vi "DSF.Engine.Interface.Builder.Read.Response.vi"(8 "error in (no error)":errorcluster, 9 "timeout in ms (0)":i32 format="%d ms", 11 "Builder Interface in":refnum<class "DSF.Engine.Interface.Builder.lvclass">) -> (0 "error out":errorcluster, 1 "empty?":bool, 2 "response":T1, 3 "Builder Interface out":refnum<class "DSF.Engine.Interface.Builder.lvclass">, 4 "# elements":u32)   [LabVIEW 2017, in "DSF.Engine.lvlib" / "DSF.Engine.Interface.Builder.lvclass"]
uses:
  DSF.Engine.Interface.Builder.lvclass
  C:/github/data-sharing-framework/dsf core/Source/Engine/Classes/Interface/DSF.Engine.Interface.lvclass
  DSF.Engine.Interface.Builder.Response Data.ctl
  DSF.Engine.Interface.Builder.Response.ctl
  DSF.Engine.Interface.lvclass/DSF.Engine.Interface.ctl
  Debug/DSF.Engine.Debug Flags.FIFO.lvclass/DSF.Engine.Debug Flags.FIFO.ctl
  Debug/DSF.Engine.Debug Flags.FIFO.Get Infinite Timeouts.vi
  Debug/DSF.Engine.Debug Flags.FIFO.lvclass
  DSF.Engine.Interface.lvclass
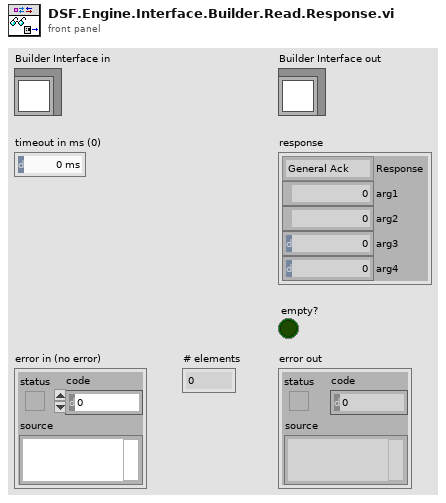
[diagram p1: front panel]
types:
  T1 = typedef "DSF.Engine.lvlib/DSF.Engine.Interface.Builder.lvclass/DSF.Engine.Interface.Builder.Response Data.ctl" = cluster{"Response":T2, "arg1":i32, "arg2":i32, "arg3":i32, "arg4":i32}
  T2 = typedef "DSF.Engine.lvlib/DSF.Engine.Interface.Builder.lvclass/DSF.Engine.Interface.Builder.Response.ctl" = enum8{"General Ack", "Initialize Complete", "Build Complete", "Parse Complete", "Shutdown Ack"}
  T3 = typedef "DSF.Engine.lvlib/DSF.Engine.Interface.lvclass/DSF.Engine.Interface.RT FIFO.Ref.16B.ctl" = refnum<k33>
  T4 = typedef "DSF.Engine.lvlib/DSF.Engine.Interface.lvclass/DSF.Engine.Interface.RT FIFO.Data.16B.ctl" = cluster{"Command":u8, "Payload":T5}
  T5 = typedef "DSF.Engine.lvlib/DSF.Engine.Interface.lvclass/DSF.Engine.Interface.RT FIFO.Payload.16B.ctl" = cluster{"arg1":u64, "arg2":u64}
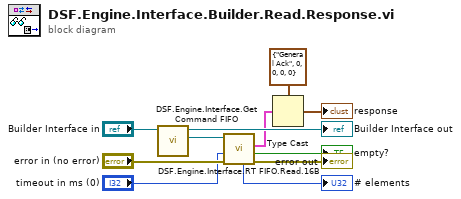
[diagram p0: block diagram]
diagram:
  n1 = call "DSF.Engine.Interface.Get Command FIFO.vi"("Interface in"="Builder Interface in") -> ("Command FIFO"=w11:T3, "Interface out"=→"Builder Interface out":refnum<class "DSF.Engine.Interface.Builder.lvclass">)  [unwired: 9 in]
  n2 = call "DSF.Engine.Interface.RT FIFO.Read.16B.vi"("error in (no error)"="error in (no error)", "timeout in ms (0)"="timeout in ms (0)", "RT FIFO in"=w11) -> ("error out"=→"error out":errorcluster, "empty?"=→"empty?":bool, "element out"=w3:T4, "# elements"=→"# elements":u32)  [unwired: 4 in, 1 out]
  n3 = Type Cast(type=T1 {"Response"=enum."General Ack", "arg1"=0, "arg2"=0, "arg3"=0, "arg4"=0} ("Plugin Response"), x=w3) -> (*(type *) &x=→"response":T1)
